vi "Creat_Traj_Config_Convert_V_internal_To_V4.vi"(11 "TrajCreateConfig V_Internal":T1 {"WayPoints"."WEIGHT" format="%13.3f"; "WayPoints"."ANGLE" format="%13.3f"; "WayPoints"."Y" format="%13.3f"; "WayPoints"."X" format="%13.3f"; "TRAJECTORY_CONFIG"."End Velocity" format="%20.4f"; "TRAJECTORY_CONFIG"."StartVelocity" format="%20.4f"; "TRAJECTORY_CONFIG"."Max Acceleration" format="%20.4f"; "TRAJECTORY_CONFIG"."MaxVelocity" format="%20.4f"}) -> (3 "TrajCreateConfig V4":T5={"Write Config File Name"=path "", "Write Config File Comment"="", "WayPoints"=[], "TRAJECTORY_CONFIG_V4"={"MaxVelocity"=0.0, "Max Acceleration"=0.0, "StartVelocity"=0.0, "End Velocity"=0.0, "Reversed"=FALSE, "DiffDrKineConstntDefined"=FALSE, "CentAcellConstntDefined"=FALSE, "DiffDrVoltConstntDefined"=FALSE, "DIFF_DRIVE_KINE_CONSTRAINT"={"Max Speed (M/S)"=0.0, "DIFF_DRIVE_KINEMATICS"={"TrackWidth_Meters"=0.0}, "Max Accel (M/S2)"=99999.0}, "CENTRIPETAL_ACCEL_CONSTRAINT"={"Max Cent Accel"=0.0}, "SwerveDrKineConstntDefined"=FALSE, "SWERVE_DRIVE_KINE_CONSTRAINT"={"Max Speed (M/S)"=0.0, "SwerveKinematics"={"NumModules"=0, "InverseKinematics"=[], "ForwardKinematics"=[], "Modules"=[], "PrevCoR"={"X"=0.0, "Y"=0.0}}}, "DIFF_DRIVE_VOLTAGE_CONSTRAINT"={"Max Voltage"=0.0, "DIFF_DRIVE_KINEMATICS"={"TrackWidth_Meters"=0.0}, "SIMPLE_MOTOR_FF"={"Ks"=0.0, "Kv"=0.0, "Ka"=0.0}}, "MECANUM_DRIVE_KINE_CONSTRAINT"={"Max Speed (M/S)"=0.0, "MECA_DRIVE_KINEMATICS"={"FrontLeft"={"X"=0.0, "Y"=0.0}, "FrontRight"={"X"=0.0, "Y"=0.0}, "RearLeft"={"X"=0.0, "Y"=0.0}, "RearRight"={"X"=0.0, "Y"=0.0}, "InverseKinematics"=[[0.0, 1.0, -1.0, 0.0], [0.0, 1.0, 1.0, 0.0], [0.0, 1.0, 1.0, 0.0], [0.0, 1.0, -1.0, 0.0]], "ForwardKinematics"=[[0.0, 1.0, -1.0, 0.0], [0.0, 1.0, 1.0, 0.0], [0.0, 1.0, 1.0, 0.0], [0.0, 1.0, -1.0, 0.0]], "PrevCoR"={"X"=0.0, "Y"=0.0}}}, "MecanumDrKineConstntDefined"=FALSE}, "FieldName"="", "Units Selector"=enum."Inches", "UseWeights"=FALSE, "IsCubic"=FALSE} {"WayPoints"."WEIGHT" format="%13.3f"; "WayPoints"."ANGLE" format="%13.3f"; "WayPoints"."Y" format="%13.3f"; "WayPoints"."X" format="%13.3f"; "TRAJECTORY_CONFIG_V4"."MECANUM_DRIVE_KINE_CONSTRAINT"."MECA_DRIVE_KINEMATICS"."PrevCoR"."Y" format="%14.3f"; "TRAJECTORY_CONFIG_V4"."MECANUM_DRIVE_KINE_CONSTRAINT"."MECA_DRIVE_KINEMATICS"."PrevCoR"."X" format="%14.3f"; "TRAJECTORY_CONFIG_V4"."MECANUM_DRIVE_KINE_CONSTRAINT"."MECA_DRIVE_KINEMATICS"."RearRight"."Y" format="%14.3f"; "TRAJECTORY_CONFIG_V4"."MECANUM_DRIVE_KINE_CONSTRAINT"."MECA_DRIVE_KINEMATICS"."RearRight"."X" format="%14.3f"; "TRAJECTORY_CONFIG_V4"."MECANUM_DRIVE_KINE_CONSTRAINT"."MECA_DRIVE_KINEMATICS"."RearLeft"."Y" format="%14.3f"; "TRAJECTORY_CONFIG_V4"."MECANUM_DRIVE_KINE_CONSTRAINT"."MECA_DRIVE_KINEMATICS"."RearLeft"."X" format="%14.3f"; "TRAJECTORY_CONFIG_V4"."MECANUM_DRIVE_KINE_CONSTRAINT"."MECA_DRIVE_KINEMATICS"."FrontRight"."Y" format="%14.3f"; "TRAJECTORY_CONFIG_V4"."MECANUM_DRIVE_KINE_CONSTRAINT"."MECA_DRIVE_KINEMATICS"."FrontRight"."X" format="%14.3f"; "TRAJECTORY_CONFIG_V4"."MECANUM_DRIVE_KINE_CONSTRAINT"."MECA_DRIVE_KINEMATICS"."FrontLeft"."Y" format="%14.3f"; "TRAJECTORY_CONFIG_V4"."MECANUM_DRIVE_KINE_CONSTRAINT"."MECA_DRIVE_KINEMATICS"."FrontLeft"."X" format="%14.3f"; "TRAJECTORY_CONFIG_V4"."MECANUM_DRIVE_KINE_CONSTRAINT"."Max Speed (M/S)" format="%20.4f"; "TRAJECTORY_CONFIG_V4"."DIFF_DRIVE_VOLTAGE_CONSTRAINT"."SIMPLE_MOTOR_FF"."Ka" format="%13.4f"; "TRAJECTORY_CONFIG_V4"."DIFF_DRIVE_VOLTAGE_CONSTRAINT"."SIMPLE_MOTOR_FF"."Kv" format="%13.4f"; "TRAJECTORY_CONFIG_V4"."DIFF_DRIVE_VOLTAGE_CONSTRAINT"."SIMPLE_MOTOR_FF"."Ks" format="%13.4f"; "TRAJECTORY_CONFIG_V4"."DIFF_DRIVE_VOLTAGE_CONSTRAINT"."DIFF_DRIVE_KINEMATICS"."TrackWidth_Meters" format="%20.4f"; "TRAJECTORY_CONFIG_V4"."DIFF_DRIVE_VOLTAGE_CONSTRAINT"."Max Voltage" format="%20.4f"; "TRAJECTORY_CONFIG_V4"."SWERVE_DRIVE_KINE_CONSTRAINT"."SwerveKinematics"."PrevCoR"."Y" format="%14.3f"; "TRAJECTORY_CONFIG_V4"."SWERVE_DRIVE_KINE_CONSTRAINT"."SwerveKinematics"."PrevCoR"."X" format="%14.3f"; "TRAJECTORY_CONFIG_V4"."SWERVE_DRIVE_KINE_CONSTRAINT"."SwerveKinematics"."Modules"."Y" format="%14.3f"; "TRAJECTORY_CONFIG_V4"."SWERVE_DRIVE_KINE_CONSTRAINT"."SwerveKinematics"."Modules"."X" format="%14.3f"; "TRAJECTORY_CONFIG_V4"."SWERVE_DRIVE_KINE_CONSTRAINT"."Max Speed (M/S)" format="%20.4f"; "TRAJECTORY_CONFIG_V4"."CENTRIPETAL_ACCEL_CONSTRAINT"."Max Cent Accel" format="%20.4f"; "TRAJECTORY_CONFIG_V4"."DIFF_DRIVE_KINE_CONSTRAINT"."Max Accel (M/S2)" format="%20.4f"; "TRAJECTORY_CONFIG_V4"."DIFF_DRIVE_KINE_CONSTRAINT"."DIFF_DRIVE_KINEMATICS"."TrackWidth_Meters" format="%20.4f"; "TRAJECTORY_CONFIG_V4"."DIFF_DRIVE_KINE_CONSTRAINT"."Max Speed (M/S)" format="%20.4f"; "TRAJECTORY_CONFIG_V4"."End Velocity" format="%20.4f"; "TRAJECTORY_CONFIG_V4"."StartVelocity" format="%20.4f"; "TRAJECTORY_CONFIG_V4"."Max Acceleration" format="%20.4f"; "TRAJECTORY_CONFIG_V4"."MaxVelocity" format="%20.4f"})   [LabVIEW 2019]
uses:
  TrajCreateConfig_V4.ctl
  <vilib>/Rock Robotics/WPI/ThirdParty/JAS_Junk/TrajLib/DISPLAY_WEIGHTED_WAYPOINT.ctl
  TrajCreateTrajConfig_V4.ctl
  <vilib>/Rock Robotics/WPI/ThirdParty/JAS_Junk/TrajLib/TRAJ_CONSTRAINT_DIIF_DRIVE_KINEMATICS.ctl
  <vilib>/Rock Robotics/WPI/ThirdParty/JAS_Junk/TrajLib/DIFF_DRIVE_KINEMATICS.ctl
  <vilib>/Rock Robotics/WPI/ThirdParty/JAS_Junk/TrajLib/TRAJ_CONSTRAINT_CENTRIPETAL_ACCEL.ctl
  <vilib>/Rock Robotics/WPI/ThirdParty/JAS_Junk/TrajLib/TRAJ_CONSTRAINT_SWERVE_DRIVE_KINEMATICS.ctl
  <vilib>/Rock Robotics/WPI/ThirdParty/JAS_Junk/TrajLib/SWERVE_DRIVE_KINEMATICS.ctl
  <vilib>/Analysis/Matrix/Datatypes/RealMatrix.ctl
  <vilib>/Rock Robotics/WPI/ThirdParty/JAS_Junk/TrajLib/TRANSLATION2D.ctl
  <vilib>/Rock Robotics/WPI/ThirdParty/JAS_Junk/TrajLib/TRAJ_CONSTRAINT_DIIF_DRIVE_VOLTAGE.ctl
  <vilib>/Rock Robotics/WPI/ThirdParty/JAS_Junk/TrajLib/SIMPLE_MOTOR_FF.ctl
  <vilib>/Rock Robotics/WPI/ThirdParty/JAS_Junk/TrajLib/TRAJ_CONSTRAINT_MECA_DRIVE_KINEMATICS.ctl
  <vilib>/Rock Robotics/WPI/ThirdParty/JAS_Junk/TrajLib/MECA_DRIVE_KINEMATICS.ctl
  TrajCreateUnitsENUM.ctl
  <vilib>/Rock Robotics/WPI/ThirdParty/JAS_Junk/TrajLib/Trajectory_Library.lvlib
  <vilib>/Analysis/Matrix/NI_Matrix.lvlib
  <vilib>/Rock Robotics/WPI/ThirdParty/JAS_Junk/TrajLib/TRAJ_CONFIG.ctl
  TrajCreateConfig__V_Internal.ctl
panel:
  # "ARRAY OF OTHER\nCONSTRAINTS \nGOES HERE.."
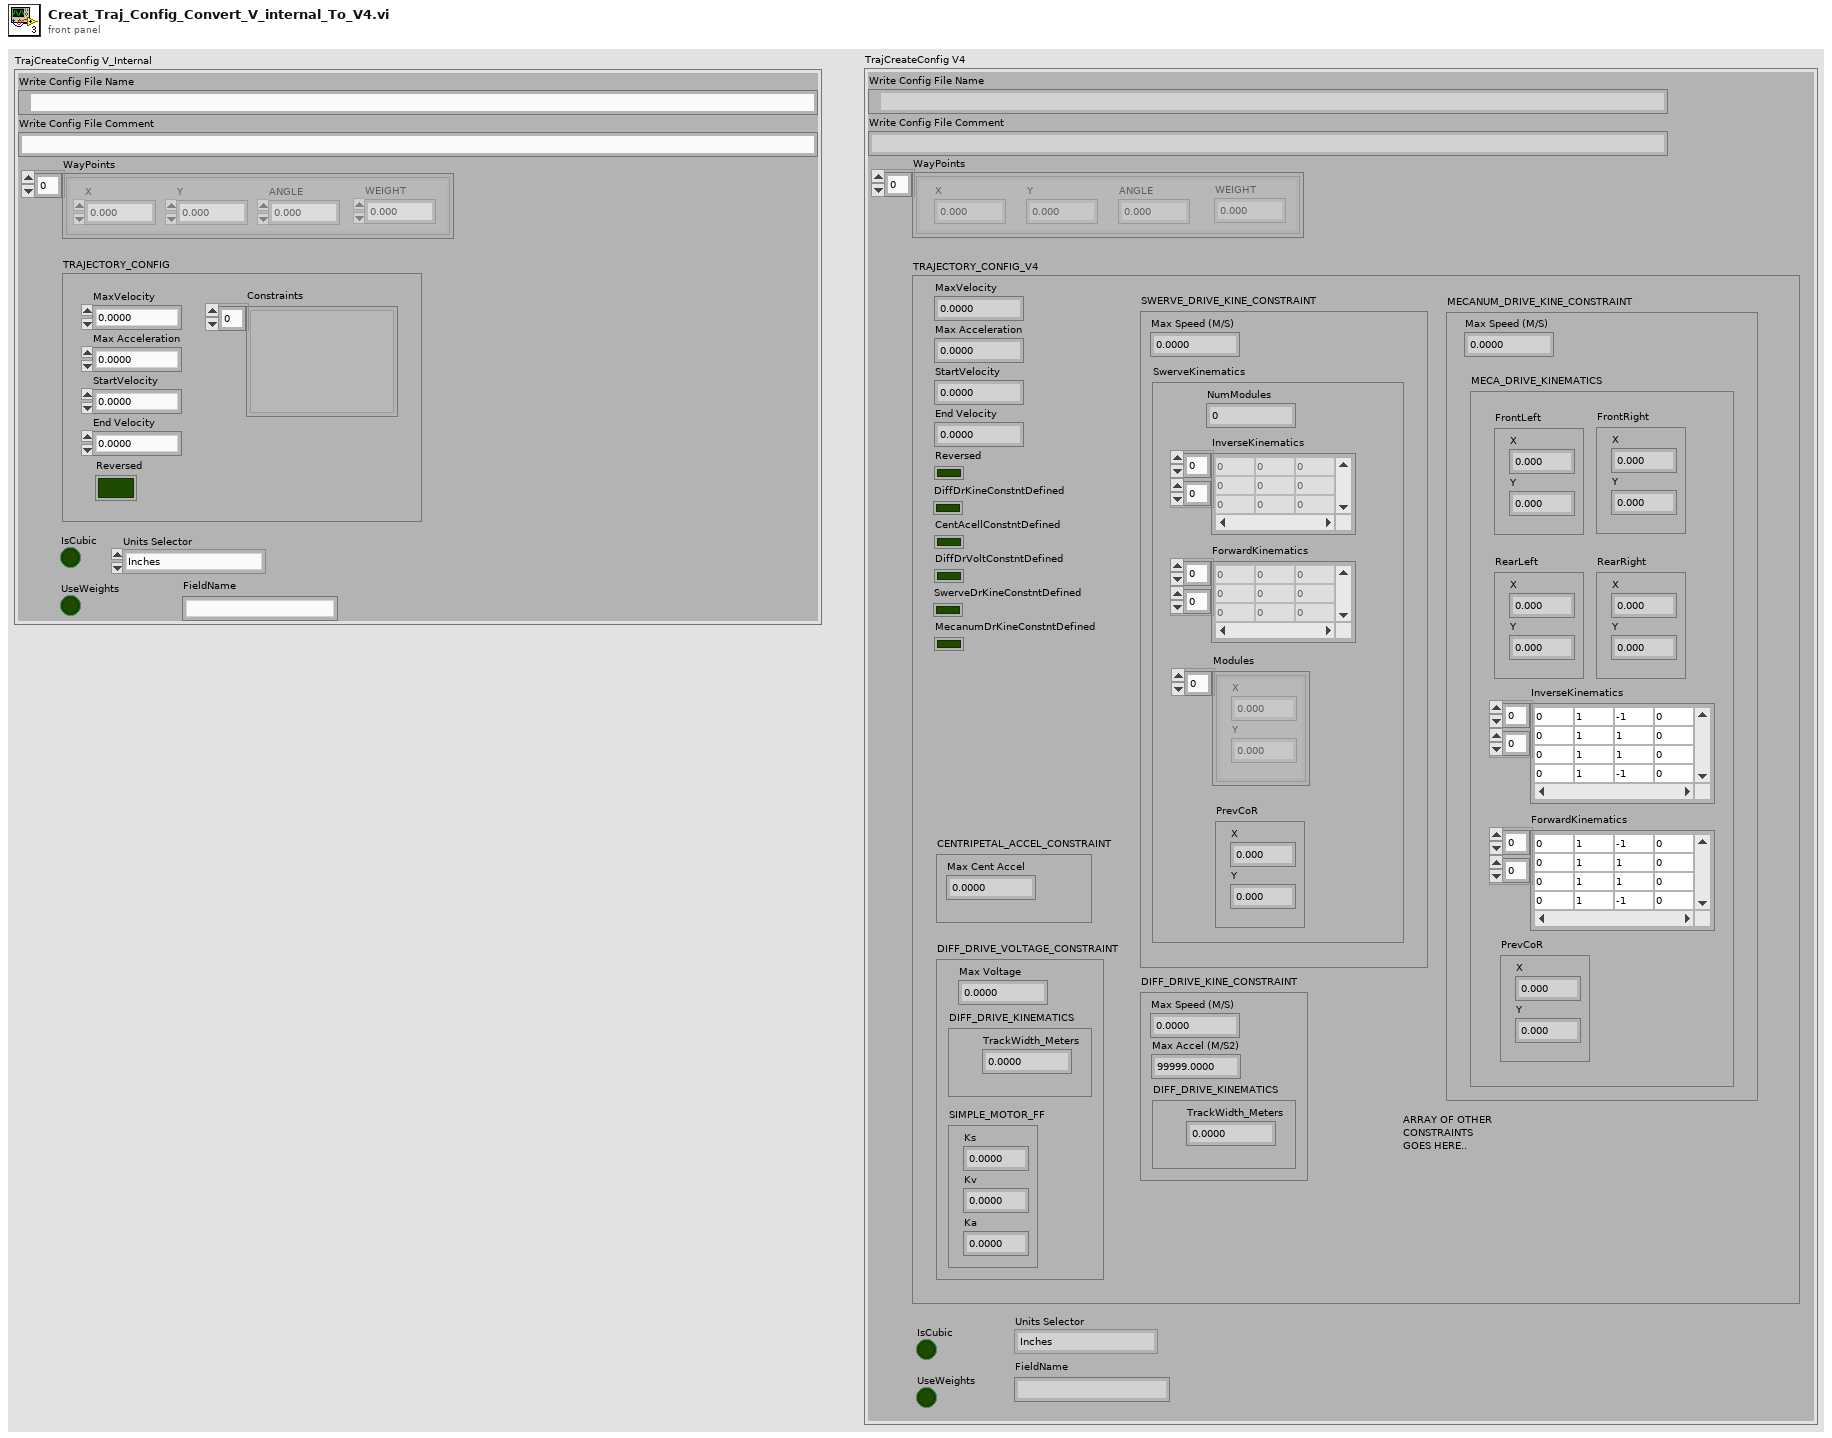
[diagram p1: front panel]
types:
  T1 = typedef "TrajCreateConfig__V_Internal.ctl" = cluster{"Write Config File Name":path, "Write Config File Comment":string, "WayPoints":T2[], "TRAJECTORY_CONFIG":T3, "IsCubic":bool, "Units Selector":T4, "UseWeights":bool, "FieldName":string}
  T2 = typedef "Trajectory_Library.lvlib/DISPLAY_WEIGHTED_WAYPOINT.ctl" = cluster{"X":dbl, "Y":dbl, "ANGLE":dbl, "WEIGHT":dbl}
  T3 = typedef "Trajectory_Library.lvlib/TRAJ_CONFIG.ctl" = cluster{"MaxVelocity":dbl, "Max Acceleration":dbl, "StartVelocity":dbl, "End Velocity":dbl, "Reversed":bool, "Constraints":variant[]}
  T4 = typedef "TrajCreateUnitsENUM.ctl" = enum16{"Inches", "Feet", "Centimeters", "Meters"}
  T5 = typedef "TrajCreateConfig_V4.ctl" = cluster{"Write Config File Name":path, "Write Config File Comment":string, "WayPoints":T2[], "TRAJECTORY_CONFIG_V4":T6, "FieldName":string, "Units Selector":T4, "UseWeights":bool, "IsCubic":bool}
  T6 = typedef "TrajCreateTrajConfig_V4.ctl" = cluster{"MaxVelocity":dbl, "Max Acceleration":dbl, "StartVelocity":dbl, "End Velocity":dbl, "Reversed":bool, "DiffDrKineConstntDefined":bool, "CentAcellConstntDefined":bool, "DiffDrVoltConstntDefined":bool, "DIFF_DRIVE_KINE_CONSTRAINT":T7, "CENTRIPETAL_ACCEL_CONSTRAINT":T9, "SwerveDrKineConstntDefined":bool, "SWERVE_DRIVE_KINE_CONSTRAINT":T10, "DIFF_DRIVE_VOLTAGE_CONSTRAINT":T14, "MECANUM_DRIVE_KINE_CONSTRAINT":T16, "MecanumDrKineConstntDefined":bool}
  T7 = typedef "Trajectory_Library.lvlib/TRAJ_CONSTRAINT_DIIF_DRIVE_KINEMATICS.ctl" = cluster{"Max Speed (M/S)":dbl, "DIFF_DRIVE_KINEMATICS":T8, "Max Accel (M/S2)":dbl}
  T8 = typedef "Trajectory_Library.lvlib/DIFF_DRIVE_KINEMATICS.ctl" = cluster{"TrackWidth_Meters":dbl}
  T9 = typedef "Trajectory_Library.lvlib/TRAJ_CONSTRAINT_CENTRIPETAL_ACCEL.ctl" = cluster{"Max Cent Accel":dbl}
  T10 = typedef "Trajectory_Library.lvlib/TRAJ_CONSTRAINT_SWERVE_DRIVE_KINEMATICS.ctl" = cluster{"Max Speed (M/S)":dbl, "SwerveKinematics":T11}
  T11 = typedef "Trajectory_Library.lvlib/SWERVE_DRIVE_KINEMATICS.ctl" = cluster{"NumModules":i32, "InverseKinematics":T12, "ForwardKinematics":T12, "Modules":T13[], "PrevCoR":T13}
  T12 = typedef "NI_Matrix.lvlib/RealMatrix.ctl" = dbl[][]
  T13 = typedef "Trajectory_Library.lvlib/TRANSLATION2D.ctl" = cluster{"X":dbl, "Y":dbl}
  T14 = typedef "Trajectory_Library.lvlib/TRAJ_CONSTRAINT_DIIF_DRIVE_VOLTAGE.ctl" = cluster{"Max Voltage":dbl, "DIFF_DRIVE_KINEMATICS":T8, "SIMPLE_MOTOR_FF":T15}
  T15 = typedef "Trajectory_Library.lvlib/SIMPLE_MOTOR_FF.ctl" = cluster{"Ks":dbl, "Kv":dbl, "Ka":dbl}
  T16 = typedef "Trajectory_Library.lvlib/TRAJ_CONSTRAINT_MECA_DRIVE_KINEMATICS.ctl" = cluster{"Max Speed (M/S)":dbl, "MECA_DRIVE_KINEMATICS":T17}
  T17 = typedef "Trajectory_Library.lvlib/MECA_DRIVE_KINEMATICS.ctl" = cluster{"FrontLeft":T13, "FrontRight":T13, "RearLeft":T13, "RearRight":T13, "InverseKinematics":T12, "ForwardKinematics":T12, "PrevCoR":T13}
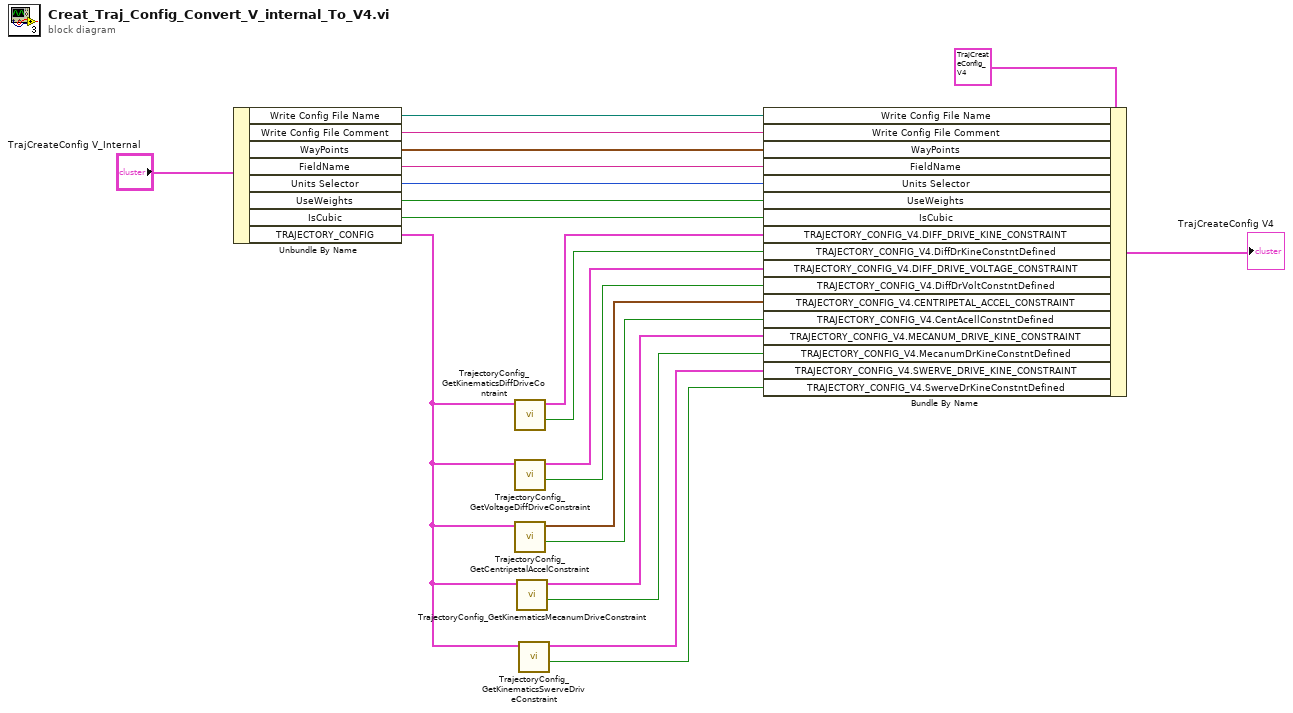
[diagram p0: block diagram]
diagram:
  n1 = Unbundle By Name("TrajCreateConfig V_Internal") -> ("Write Config File Name"=w20:path, "Write Config File Comment"=w19:string, "WayPoints"=w18:T2[], "FieldName"=w17:string, "Units Selector"=w16:T4, "UseWeights"=w15:bool, "IsCubic"=w14:bool, "TRAJECTORY_CONFIG"=w11:T3)
  n2 = call <vilib>:"TrajectoryConfig_GetKinematicsDiffDriveContraint.vi"("inTRAJECTORY_CONFIG"=w11) -> ("Constraint Exists"=w9:bool, "Diff Drive Kinematics Constraint"=w10:T7)  [unwired: 9 in]
  n3 = call <vilib>:"TrajectoryConfig_GetVoltageDiffDriveConstraint.vi"("inTRAJECTORY_CONFIG"=w11) -> ("Constraint Exists"=w7:bool, "Differential Drive Voltage Constraint"=w8:T14)  [unwired: 9 in]
  n4 = call <vilib>:"TrajectoryConfig_GetCentripetalAccelConstraint.vi"("inTRAJECTORY_CONFIG"=w11) -> ("Constraint Exists"=w5:bool, "Centripital Accleration Constraint"=w6:T9)  [unwired: 9 in]
  n5 = call <vilib>:"TrajectoryConfig_GetKinematicsMecanumDriveConstraint.vi"("inTRAJECTORY_CONFIG"=w11) -> ("Constraint Exists"=w3:bool, "Mecanum Drive Kinematics Constraint"=w4:T16)  [unwired: 9 in]
  n6 = call <vilib>:"TrajectoryConfig_GetKinematicsSwerveDriveConstraint.vi"("inTRAJECTORY_CONFIG"=w11) -> ("Constraint Exists"=w1:bool, "Swerver Drive Kinematics Constraint"=w2:T10)  [unwired: 9 in]
  n7 = Bundle By Name(cluster=T5 {"Write Config File Name"=path "", "Write Config File Comment"="", "WayPoints"=[], "TRAJECTORY_CONFIG_V4"={"MaxVelocity"=0.0, "Max Acceleration"=0.0, "StartVelocity"=0.0, "End Velocity"=0.0, "Reversed"=FALSE, "DiffDrKineConstntDefined"=FALSE, "CentAcellConstntDefined"=FALSE, "DiffDrVoltConstntDefined"=FALSE, "DIFF_DRIVE_KINE_CONSTRAINT"={"Max Speed (M/S)"=0.0, "DIFF_DRIVE_KINEMATICS"={"TrackWidth_Meters"=0.0}, "Max Accel (M/S2)"=99999.0}, "CENTRIPETAL_ACCEL_CONSTRAINT"={"Max Cent Accel"=0.0}, "SwerveDrKineConstntDefined"=FALSE, "SWERVE_DRIVE_KINE_CONSTRAINT"={"Max Speed (M/S)"=0.0, "SwerveKinematics"={"NumModules"=0, "InverseKinematics"=[], "ForwardKinematics"=[], "Modules"=[], "PrevCoR"={"X"=0.0, "Y"=0.0}}}, "DIFF_DRIVE_VOLTAGE_CONSTRAINT"={"Max Voltage"=0.0, "DIFF_DRIVE_KINEMATICS"={"TrackWidth_Meters"=0.0}, "SIMPLE_MOTOR_FF"={"Ks"=0.0, "Kv"=0.0, "Ka"=0.0}}, "MECANUM_DRIVE_KINE_CONSTRAINT"={"Max Speed (M/S)"=0.0, "MECA_DRIVE_KINEMATICS"={"FrontLeft"={"X"=0.0, "Y"=0.0}, "FrontRight"={"X"=0.0, "Y"=0.0}, "RearLeft"={"X"=0.0, "Y"=0.0}, "RearRight"={"X"=0.0, "Y"=0.0}, "InverseKinematics"=[[0.0, 1.0, -1.0, 0.0], [0.0, 1.0, 1.0, 0.0], [0.0, 1.0, 1.0, 0.0], [0.0, 1.0, -1.0, 0.0]], "ForwardKinematics"=[[0.0, 1.0, -1.0, 0.0], [0.0, 1.0, 1.0, 0.0], [0.0, 1.0, 1.0, 0.0], [0.0, 1.0, -1.0, 0.0]], "PrevCoR"={"X"=0.0, "Y"=0.0}}}, "MecanumDrKineConstntDefined"=FALSE}, "FieldName"="", "Units Selector"=enum."Inches", "UseWeights"=FALSE, "IsCubic"=FALSE} ("TrajCreateConfig"), "Write Config File Name"=w20, "Write Config File Comment"=w19, "WayPoints"=w18, "FieldName"=w17, "Units Selector"=w16, "UseWeights"=w15, "IsCubic"=w14, "TRAJECTORY_CONFIG_V4.DIFF_DRIVE_KINE_CONSTRAINT"=w10, "TRAJECTORY_CONFIG_V4.DiffDrKineConstntDefined"=w9, "TRAJECTORY_CONFIG_V4.DIFF_DRIVE_VOLTAGE_CONSTRAINT"=w8, "TRAJECTORY_CONFIG_V4.DiffDrVoltConstntDefined"=w7, "TRAJECTORY_CONFIG_V4.CENTRIPETAL_ACCEL_CONSTRAINT"=w6, "TRAJECTORY_CONFIG_V4.CentAcellConstntDefined"=w5, "TRAJECTORY_CONFIG_V4.MECANUM_DRIVE_KINE_CONSTRAINT"=w4, "TRAJECTORY_CONFIG_V4.MecanumDrKineConstntDefined"=w3, "TRAJECTORY_CONFIG_V4.SWERVE_DRIVE_KINE_CONSTRAINT"=w2, "TRAJECTORY_CONFIG_V4.SwerveDrKineConstntDefined"=w1) -> (→"TrajCreateConfig V4":T5)
